vi "DecimalDegreesToInches.vi"(2 "Longitude":dbl, 3 "Latitude":dbl) -> (0 "X":dbl, 1 "Y":dbl)   [LabVIEW 2010]
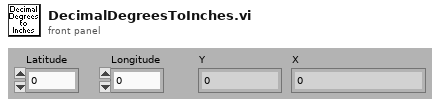
[diagram p1: front panel]
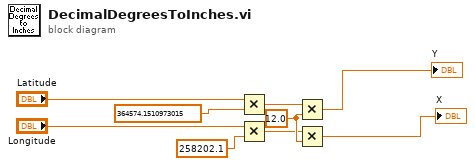
[diagram p0: block diagram]
diagram:
  w6 = 12.0 ("x")
  n1 = Multiply(x="Latitude", y=364574.1510973015 ("x")) -> (x*y=w3:dbl)
  n2 = Multiply(x="Longitude", y=258202.1 ("x")) -> (x*y=w5:dbl)
  n3 = Multiply(x=w3, y=w6) -> (x*y=→"Y":dbl)
  n4 = Multiply(x=w5, y=w6) -> (x*y=→"X":dbl)
